vi "CompareGaitTime.vi"(8 "Min Swing Time in ms (100)":u32=100, 9 "Min Stance Time in ms (100)":u32=100, 11 "GaitPhase":T1=enum."ToeOff") -> (3 "Minimum Time Passed":bool)   [LabVIEW 2016, in "ForceField.lvclass"]
uses:
  ForceField.lvclass
  TypeDef/GaitPhase.ctl
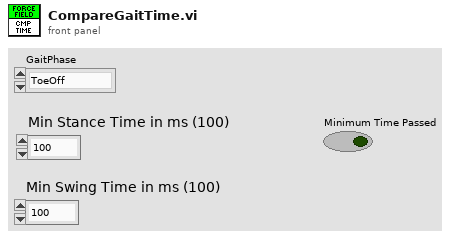
[diagram p1: front panel]
types:
  T1 = typedef "ForceField.lvclass/GaitPhase.ctl" = enum16{"HeelStrk", "Stance", "ToeOff", "Swing"}
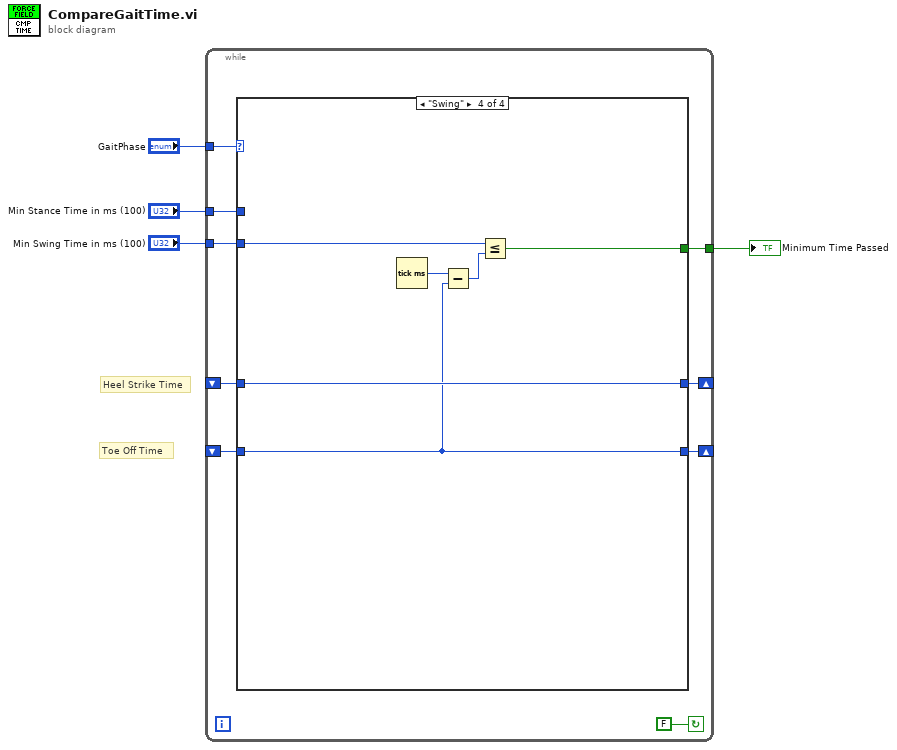
[diagram p0: block diagram]
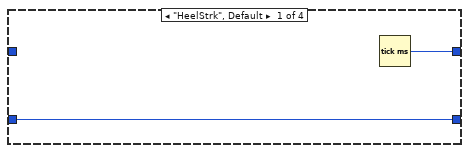
[diagram p2: hidden frame]
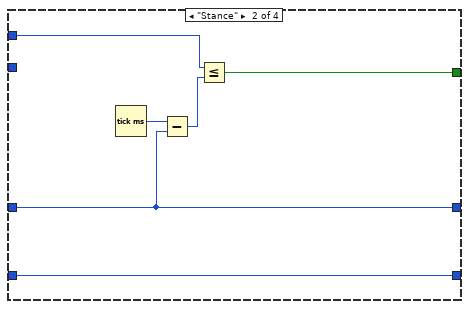
[diagram p3: hidden frame]
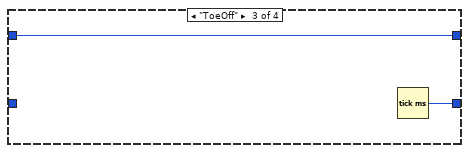
[diagram p4: hidden frame]
diagram:
  # "Toe Off Time"
  # "Heel Strike Time"
  n1 = while {
    tunnel: [w13] -> w4
    tunnel: "GaitPhase" -> [w12]
    shift-right: [w11] -> _
    shift-left: _ -> [w9]
    shift-right: [w10] -> _
    shift-left: _ -> [w8]
    tunnel: "Min Swing Time in ms (100)" -> [w7]
    tunnel: "Min Stance Time in ms (100)" -> [w6]
    stop <- FALSE continue-if-true
    n2 = case shown="\"Swing\"" w12 {
      tunnel: [_ w21 _ w27] -> w13
      tunnel: [w15 w17 w22 w26] -> w11
      tunnel: [w14 w18 w23 w25] -> w10
      tunnel: w9 -> [_ w17 w22 w26]
      tunnel: w8 -> [w14 w18 _ w25]
      tunnel: w7 -> [_ _ _ w24]
      tunnel: w6 -> [_ w16 _ _]
      frame "HeelStrk", Default {
        n3 = Tick Count (ms)() -> (millisecond timer value=w15:u32)
      }
      frame "Stance" {
        n4 = Tick Count (ms)() -> (millisecond timer value=w19:u32)
        n5 = Subtract(x=w19, y=w17) -> (x-y=w20:u32)
        n6 = Less Or Equal?(x=w16, y=w20) -> (x <= y?=w21:bool)
      }
      frame "ToeOff" {
        n7 = Tick Count (ms)() -> (millisecond timer value=w23:u32)
      }
      frame "Swing" {
        n8 = Tick Count (ms)() -> (millisecond timer value=w28:u32)
        n9 = Subtract(x=w28, y=w25) -> (x-y=w29:u32)
        n10 = Less Or Equal?(x=w24, y=w29) -> (x <= y?=w27:bool)
      }
    }
  }
  "Minimum Time Passed" <- w4
